vi "Write Pulse Rectifier Recipe to ListBox.vi"(4 "Right AmpMins":dbl[](array[numeric]), 5 "Left AmpMins":dbl[](array[numeric]), 6 "Right Amps":dbl[](array[numeric]), 7 "Left Amps":dbl[](array[numeric]), 8 "error in (no error)":errorcluster, 10 "Number Steps":i32, 11 "ListBox":refnum<vi>) -> (0 "error out":errorcluster)   [LabVIEW 2019]
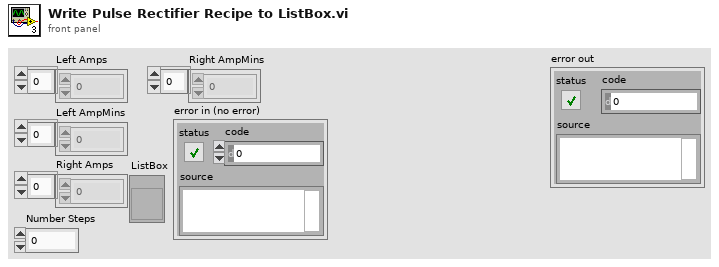
[diagram p1: front panel]
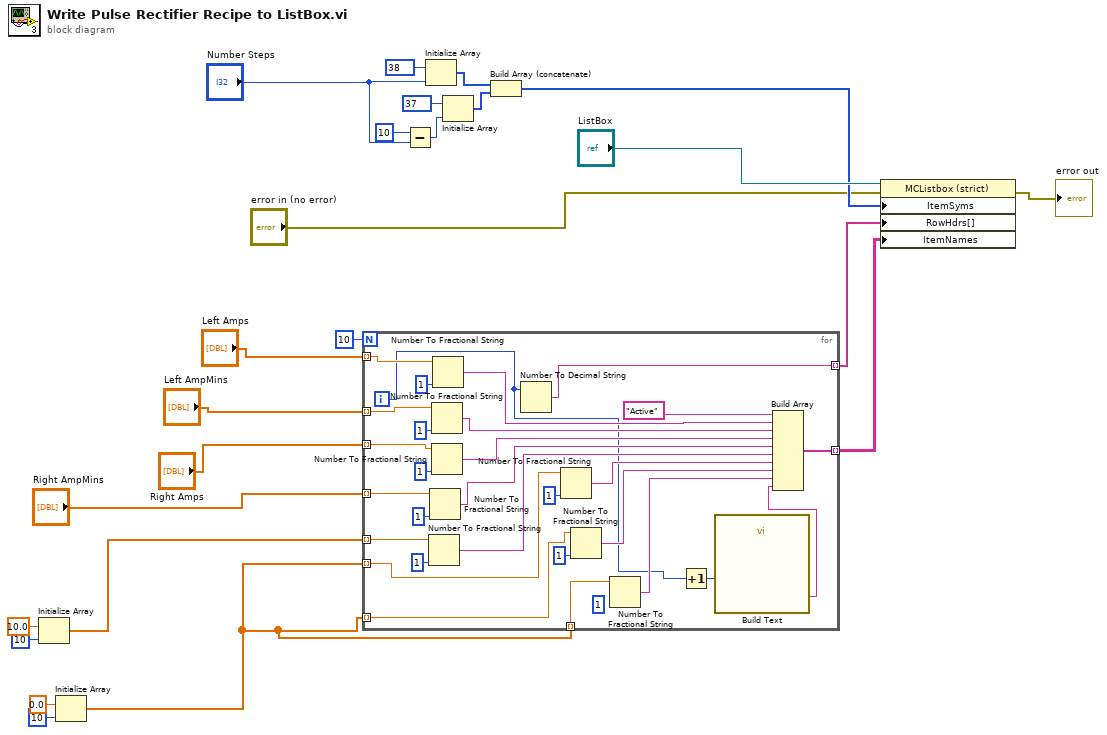
[diagram p0: block diagram]
diagram:
  n1 = Initialize Array(10.0 ("element"), 10 ("dimension size")) -> (w5:dbl[])
  n2 = Initialize Array(0.0 ("element"), 10 ("dimension size")) -> (w2:dbl[])
  n3 = for {
    N: 10 -> [_]
    tunnel: "Left Amps" -> [w48] mode=indexing
    tunnel: "Left AmpMins" -> [w47] mode=indexing
    tunnel: "Right Amps" -> [w46] mode=indexing
    tunnel: "Right AmpMins" -> [w45] mode=indexing
    tunnel: w5 -> [w44] mode=indexing
    tunnel: [w39] -> w9 mode=indexing
    tunnel: w2 -> [w34] mode=indexing
    tunnel: w2 -> [w33] mode=indexing
    tunnel: w2 -> [w32] mode=indexing
    tunnel: [w28] -> w1 mode=indexing
    i -> [w25]
    (unwired) i16 1 ("precision (6)")
    n4 = Number To Fractional String(number=w44, precision (6)=i16 1) -> (F-format string=w35:string)  [unwired: 2 in]
    n5 = Number To Fractional String(number=w45, precision (6)=i16 1) -> (F-format string=w36:string)  [unwired: 2 in]
    n6 = Number To Fractional String(number=w47, precision (6)=i16 1) -> (F-format string=w38:string)  [unwired: 2 in]
    n7 = Number To Fractional String(number=w46, precision (6)=i16 1) -> (F-format string=w37:string)  [unwired: 2 in]
    n8 = Number To Fractional String(number=w48, precision (6)=i16 1) -> (F-format string=w40:string)  [unwired: 2 in]
    n9 = Number To Decimal String(number=w25) -> (decimal integer string=w39:string)  [unwired: 1 in]
    n10 = Number To Fractional String(number=w34, precision (6)=i16 1) -> (F-format string=w31:string)  [unwired: 2 in]
    n11 = Number To Fractional String(number=w33, precision (6)=i16 1) -> (F-format string=w30:string)  [unwired: 2 in]
    n12 = Number To Fractional String(number=w32) -> (F-format string=w29:string)  [unwired: 3 in]
    n13 = Increment(x=w25) -> (x+1=w26:i32)
    n14 = call "Build Text"("d"=w26) -> ("Result"=w27:string)  [unwired: 13 in, 1 out]
    n15 = Build Array("Active", w40, w38, w37, w36, w35, w31, w30, w29, w27) -> (w28:string[])
  }
  n16 = Subtract(x=10, y="Number Steps") -> (x-y=w22:i32)
  n17 = Initialize Array(38, "Number Steps") -> (w21:i32[])
  n18 = Initialize Array(37, w22) -> (w20:i32[])
  n19 = Build Array (concatenate)(w21, w20) -> (w16:i32[])
  n20 = property class="MCListbox (strict)"(reference="ListBox", error in="error in (no error)", "ItemSyms"=w16, "RowHdrs[]"=w9, "ItemNames"=w1) -> (error out=→"error out":errorcluster)  [unwired: 1 out]
